vi "user name and password.vi"() -> ()   [LabVIEW 2018]
panel:
  in  "DATE":string
  in  "PASSWORD":string
  in  "USERNAME":string
  # "BOOK YOUR TICKET"
  # "IRCTC"
  # "FIND YOUR\n   TRAINS"
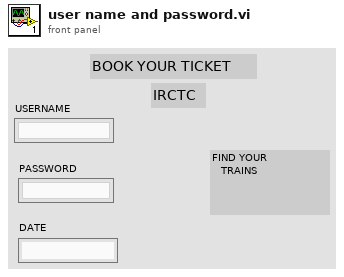
[diagram p1: front panel]
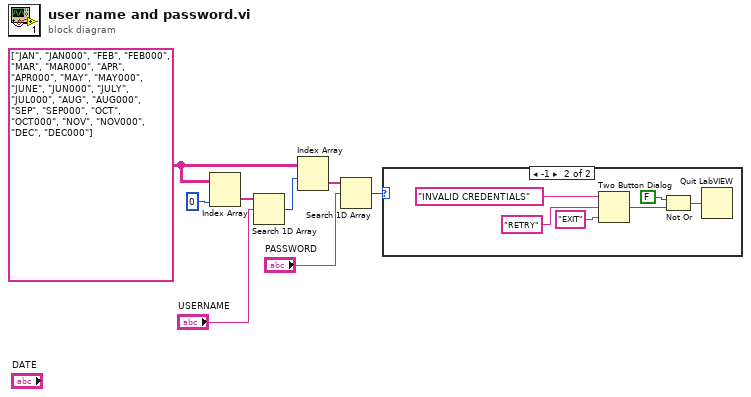
[diagram p0: block diagram]
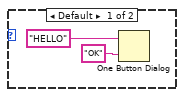
[diagram p2: hidden frame]
diagram:
  w8 = string[][] [["JAN", "JAN000"], ["FEB", "FEB000"], ["MAR", "MAR000"], ["APR", "APR000"], ["MAY", "MAY000"], ["JUNE", "JUN000"], ["JULY", "JUL000"], ["AUG", "AUG000"], ["SEP", "SEP000"], ["OCT", "OCT000"], ["NOV", "NOV000"], ["DEC", "DEC000"]]
  n1 = Index Array(array=w8, index (col)=0 ("disabled index (col)")) -> (element=w5:string[])  [unwired: 1 in]
  n2 = Search 1D Array(1D array=w5, element="USERNAME") -> (index of element=w2:i32)  [unwired: 1 in]
  n3 = Index Array(array=w8, index (row)=w2) -> (element=w3:string[])  [unwired: 1 in]
  n4 = Search 1D Array(1D array=w3, element="PASSWORD") -> (index of element=w1:i32)  [unwired: 1 in]
  n5 = case shown="-1" w1 {
    frame Default {
      n6 = One Button Dialog(message="HELLO", button name ("OK")="OK") -> ()  [unwired: 1 out]
    }
    frame -1 {
      n7 = Two Button Dialog(message="INVALID CREDENTIALS", 1:"EXIT" ("F button name (\"Cancel\")"), 2:"RETRY" ("T button name (\"OK\")")) -> (T button?=w11:bool)
      n8 = Not Or(1:w11, 2:FALSE ("x")) -> (0:w13:bool)
      n9 = Quit LabVIEW(quit? (T)=w13) -> ()
    }
  }
